vi "output.vi"(8 "error in":errorcluster, 10 "output data":T1, 11 "module in":refnum<class "TBM module execution interface.lvclass">) -> (0 "error out":errorcluster, 2 "output allocation":T1, 3 "module out":refnum<class "TBM module execution interface.lvclass">)   [LabVIEW 2013, in "TBM module execution interface.lvclass"]
doc: "Provides an interface for writing data to a module at runtime. While this interface performs no operations, a child should provide an override which may write to any open sessions, references, or interfaces."
uses:
  TBM module execution interface.lvclass
  <vilib>/NI/Tag Bus/table/data table.ctl
  root configuration/TBM configuration.lvclass
  <vilib>/NI/Tag Bus/table/data table.lvlib
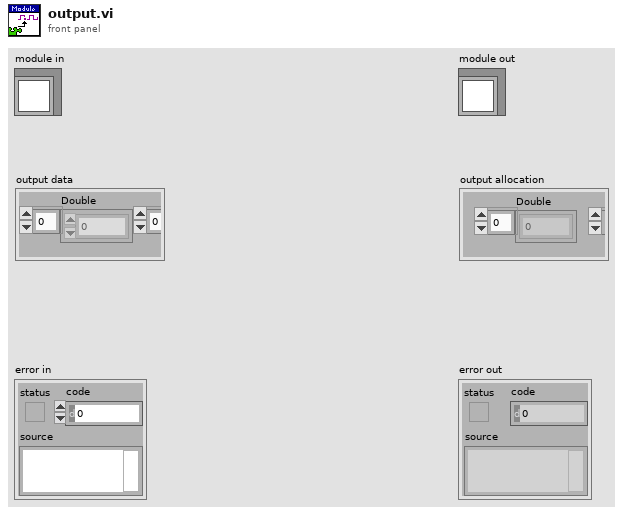
[diagram p1: front panel]
types:
  T1 = typedef "tag bus.lvlib/data table.lvlib/data table.ctl" = cluster{"Double":dbl[], "Single":sgl[], "I64":i64[], "I32":i32[], "I16":i16[], "I8":i8[], "U64":u64[], "U32":u32[], "U16":u16[], "U8":u8[], "Boolean":bool[], "String":string[], "Array of Double":cluster{"DBL Array":dbl[]}[], "Array of Single":cluster{"SGL Array":sgl[]}[], "Array of I64":cluster{"I64 Array":i64[]}[], "Array of I32":cluster{"I32 Array":i32[]}[], "Array of I16":cluster{"I16 Array":i16[]}[], "Array of I8":cluster{"I8 Array":i8[]}[], "Array of U64":cluster{"U64 Array":u64[]}[], "Array of U32":cluster{"U32 Array":u32[]}[], "Array of U16":cluster{"U16 Array":u16[]}[], "Array of U8":cluster{"U8 Array":u8[]}[], "Array of Boolean":cluster{"Boolean Array":bool[]}[], "Array of String":cluster{"String Array":string[]}[]}
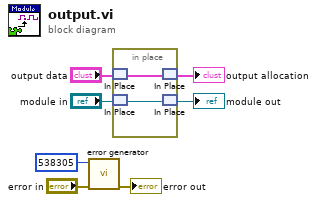
[diagram p0: block diagram]
diagram:
  n1 = call "error generator.vi"("error in"="error in", "error code (0)"=538305) -> ("error out"=→"error out":errorcluster)  [unwired: 9 in]
  n2 = in-place {
    n3 = in-place-match #1("output data") -> (w9:T1)
    n4 = in-place-match #2("module in") -> (w8:refnum<class "TBM module execution interface.lvclass">)
    n5 = in-place-match #1(w9) -> (→"output allocation":T1)
    n6 = in-place-match #2(w8) -> (→"module out":refnum<class "TBM module execution interface.lvclass">)
  }
